vi "Get Lines in String- Control.vi"() -> ()   [LabVIEW 2017]
panel:
  in  "correction":u32=13
  out "Lines":i32
  in  "desired font(Application)":T1(ring)=enum."Application Font"
  in  "[user-specified font]":T2
  in  "String":string="aaaa aaaaa aaaaa aaaaa bbbbb bbbbb bbbbb bbbbb ccccc ccccc ccccc ccccc ddddd ddddd ddddd ddddd abcdefghijklmnopqrstuvwxyz"
  # "Correction means width of String- Control\nminus borders (left & right) \nminus some Pixels in Text- Area"
  # "To determine the actual width of Text-Area the Control should\nbe resized pixel by pixel until a line changes wrapping. Then\nthe width of that wrapped line can be measured with the \nscreenshot of the String control and a graphic program.\nThe difference between the controls width and the line width\nis the correction.\nWhen this control is resized from 154 to 155 pixel width, the third\nline changes wrapping."
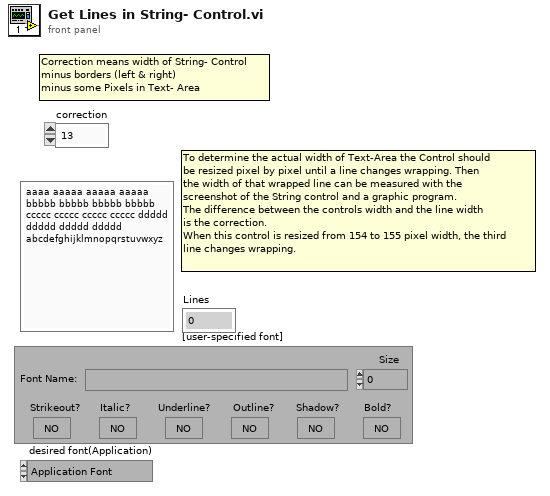
[diagram p1: front panel]
types:
  T1 = enum16{"User-specified Font", "Application Font", "System Font", "Dialog Font"}
  T2 = cluster{"Font Name:":string, "Size":i16, "Strikeout?":bool, "Italic?":bool, "Underline?":bool, "Outline?":bool, "Shadow?":bool, "Bold?":bool}
  T3 = cluster{"left":i16, "top":i16, "right":i16, "bottom":i16}
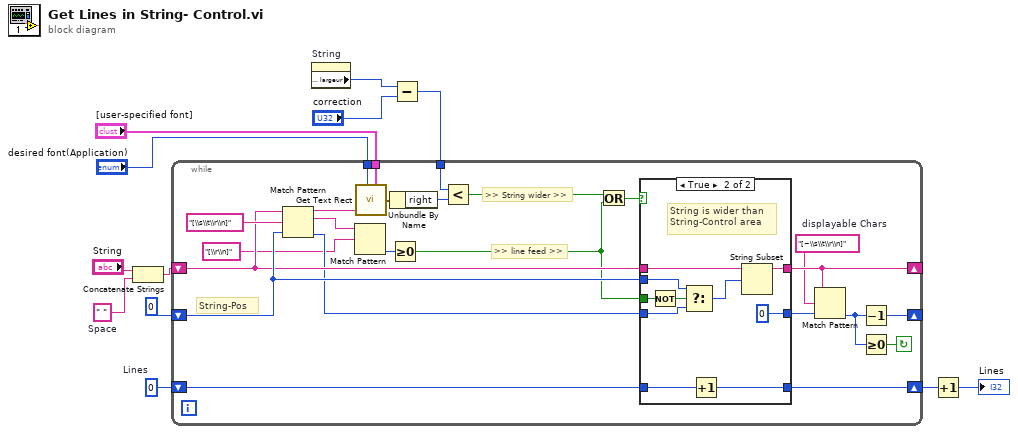
[diagram p0: block diagram]
diagram:
  w1 = " "  # Space
  w9 = 0  # Lines
  n1 = Concatenate Strings("String", w1) -> (w2:string)
  n2 = property on="String" class="Str"() -> ("Taille : largeur"=w12:u32)  [unwired: 2 in, 2 out]
  n3 = Subtract(x=w12, y="correction") -> (x-y=w4:u32)
  n4 = while {
    shift-right: [w25] -> _
    shift-left: w2 -> [w22]
    shift-right: [w23] -> _
    shift-left: 0 ("offset (0)") -> [w29]
    shift-right: [w27] -> w6
    shift-left: w9 -> [w28]
    tunnel: w4 -> [w30]
    tunnel: "desired font(Application)" -> [w34]
    tunnel: "[user-specified font]" -> [w33]
    stop <- w18 continue-if-true
    w24 = "[~\\s\\t\\r\\n]"  # displayable Chars
    # ">> line feed >>"
    # ">> String wider >>"
    # "String-Pos"
    n5 = Match Pattern(string=w22, regular expression="[\\s\\t\\r\\n]", offset (0)=w29) -> (before substring=w35:string, match substring=w16:string, offset past match=w21:i32)  [unwired: 1 out]
    n6 = Match Pattern(string=w16, regular expression="[\\r\\n]") -> (offset past match=w14:i32)  [unwired: 1 in, 3 out]
    n7 = call <vilib>:"Get Text Rect.vi"("desired font(Application)"=w34, "text"=w35, "[user-specified font]"=w33) -> ("rect"=w32:T3)  [unwired: 6 in]
    n8 = Unbundle By Name(w32) -> ("right"=w31:i16)
    n9 = Greater Or Equal To 0?(x=w14) -> (x >= 0?=w13:bool)
    n10 = Less?(x=w30, y=w31) -> (x < y?=w20:bool)
    n11 = Or(x=w20, y=w13) -> (x .or. y?=w15:bool)
    n12 = case shown="True" w15 {
      tunnel: w22 -> [w39 w49]
      tunnel: w29 -> [_ w41]
      tunnel: w28 -> [w38 w47]
      tunnel: [w39 w48] -> w25
      tunnel: [w38 w46] -> w27
      tunnel: [w37 0] -> w26
      tunnel: w21 -> [w37 w42]
      tunnel: w13 -> [_ w44]
      frame False {
      }
      frame True {
        # "String is wider than\nString-Control area"
        n13 = Not(x=w44) -> (.not. x?=w43:bool)
        n14 = Select(t=w41, s=w43, f=w42) -> (s? t:f=w40:i32)
        n15 = Increment(x=w47) -> (x+1=w46:i32)
        n16 = String Subset(string=w49, offset (0)=w40) -> (substring=w48:string)  [unwired: 1 in]
      }
    }
    n17 = Match Pattern(string=w25, regular expression=w24, offset (0)=w26) -> (offset past match=w19:i32)  [unwired: 3 out]
    n18 = Decrement(x=w19) -> (x-1=w23:i32)
    n19 = Greater Or Equal To 0?(x=w19) -> (x >= 0?=w18:bool)
  }
  n20 = Increment(x=w6) -> (x+1=→"Lines":i32)
